vi "parse_xml.vi"(8 "error in (no error)":errorcluster, 11 "XML File Path":path) -> (0 "error out":errorcluster, 3 "raw_data []":T1(array[cluster]))   [LabVIEW 2015, in "lv-unit-conversion.lvlib"]
uses:
  lv-unit-conversion.lvlib
  _controls/error.ctl
  <vilib>/xml/Load XML File.vi
  <vilib>/xml/Close Reference(Node).vi
  <vilib>/xml/NI_XML.lvlib
  <resource>/objmgr/DOMUserDefRef.rc
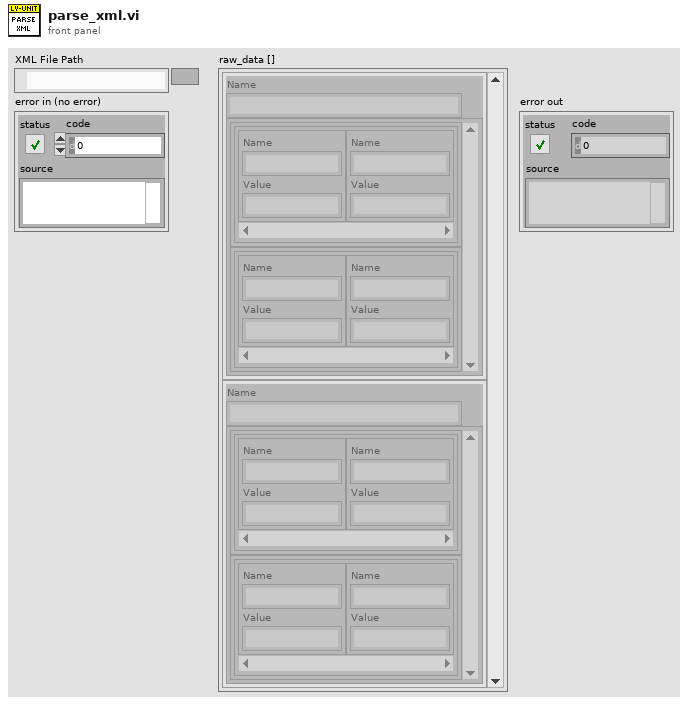
[diagram p1: front panel]
types:
  T1 = cluster{"Name":string, cluster{cluster{"Name":string, "Value":string}[]}[]}[]
  T2 = typedef "lv-unit-conversion.lvlib/error.ctl" = enum16{"<lv-unit-conversion_error>", "unit_not_found", "xml_parser", "<null>"}
  T3 = cluster{cluster{"Name":string, "Value":string}[]}
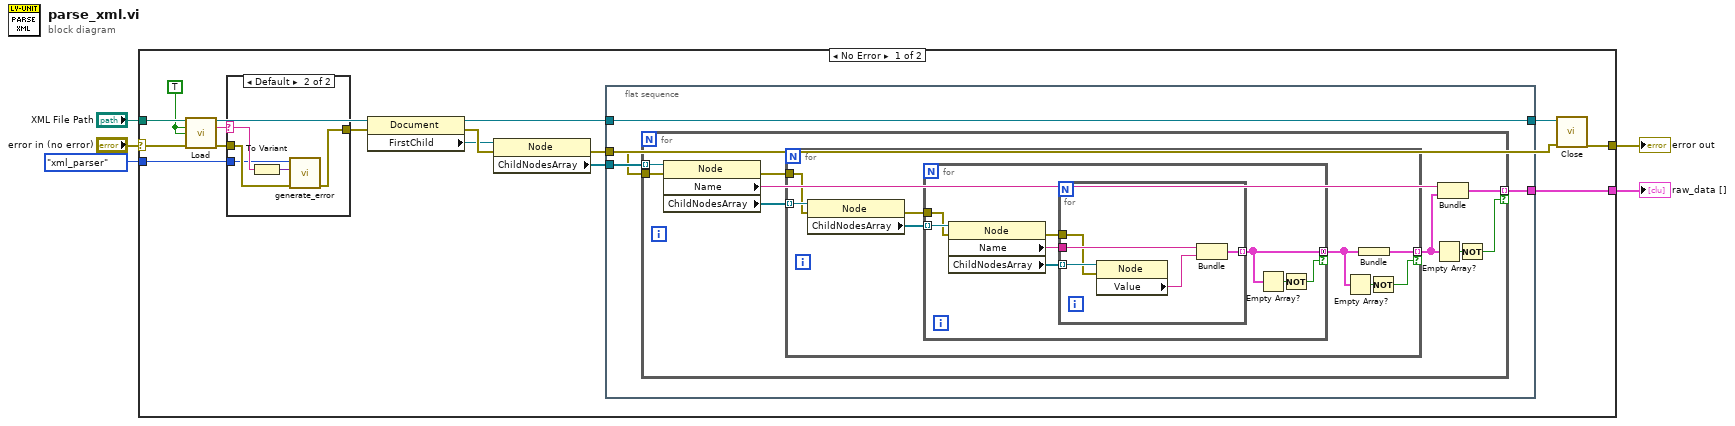
[diagram p0: block diagram]
diagram:
  n1 = case shown="No Error" "error in (no error)" {
    selector: "error in (no error)" -> [w10 w62]
    tunnel: "XML File Path" -> [w21 _]
    tunnel: [w15 _] -> w4
    tunnel: [w12 w62] -> w3
    tunnel: error."xml_parser" ("error") -> [w6 _]
    frame No Error {
      w20 = TRUE ("process namespaces (False)")
      n2 = call-poly <vilib>:"Load.vi"("path to XML document"=w21, "process namespaces (False)"=w20, "process schema (False)"=w20, "error in (no error)"=w10) -> ("DOM document out"=w19:refnum<k20>, "parse errors"=w9:string, "error out"=w8:errorcluster)  [unwired: 9 in]
      n3 = case shown="Default" w9 {
        selector: w9 -> [_ w27]
        tunnel: w8 -> [w22 w26]
        tunnel: [w22 w25] -> w7
        tunnel: w6 -> [_ w24]
        frame "" {
        }
        frame Default {
          n4 = To Variant(anything=w27) -> (Variant=w23:variant)
          n5 = call "generate_error.vi"("error in (no error)"=w26, "data"=w23, "error"=w24) -> ("error out"=w25:errorcluster)  [unwired: 8 in]
        }
      }
      n6 = property class="Document"(reference=w19, error in=w7) -> (reference out=w14:refnum<k20>, error out=w17:errorcluster, "FirstChild"=w16:refnum<k20>)
      n7 = property class="Node"(reference=w16, error in=w17) -> (error out=w11:errorcluster, "ChildNodesArray"=w18:refnum<k20>[])  [unwired: 1 out]
      n8 = flat-sequence {
        tunnel: w18 -> [w31]
        tunnel: [w30] -> w15
        tunnel: w14 -> [w29]
        tunnel: [w29] -> w13
        tunnel: w11 -> [w28]
        frame #0 {
          n9 = for {
            tunnel: w31 -> [w40] mode=indexing
            tunnel: [w39] -> w30 mode=indexing if=w36
            tunnel: w28 -> [w35]
            n10 = property class="Node"(reference=w40, error in=w35) -> (error out=w32:errorcluster, "Name"=w33:string, "ChildNodesArray"=w34:refnum<k20>[])  [unwired: 1 out]
            n11 = for {
              tunnel: w34 -> [w48] mode=indexing
              tunnel: [w44] -> w37 mode=indexing if=w45
              tunnel: w32 -> [w42]
              n12 = property class="Node"(reference=w48, error in=w42) -> (error out=w41:errorcluster, "ChildNodesArray"=w47:refnum<k20>[])  [unwired: 1 out]
              n13 = for {
                tunnel: w47 -> [w56] mode=indexing
                tunnel: [w52] -> w43 mode=concatenating if=w51
                tunnel: w41 -> [w50]
                n14 = property class="Node"(reference=w56, error in=w50) -> (error out=w49:errorcluster, "Name"=w54:string, "ChildNodesArray"=w55:refnum<k20>[])  [unwired: 1 out]
                n15 = for {
                  tunnel: w55 -> [w61] mode=indexing
                  tunnel: w54 -> [w58]
                  tunnel: [w59] -> w52 mode=indexing
                  tunnel: w49 -> [w57]
                  n16 = property class="Node"(reference=w61, error in=w57) -> ("Value"=w60:string)  [unwired: 2 out]
                  n17 = Bundle("Name"=w58, "Value"=w60) -> (w59:cluster{"Name":string, "Value":string})  [unwired: 1 in]
                }
                n18 = Empty Array?(array=w52) -> (empty?=w53:bool)
                n19 = Not(x=w53) -> (.not. x?=w51:bool)
              }
              n20 = Empty Array?(array=w43) -> (empty?=w46:bool)
              n21 = Bundle(w43) -> (w44:T3)  [unwired: 1 in]
              n22 = Not(x=w46) -> (.not. x?=w45:bool)
            }
            n23 = Empty Array?(array=w37) -> (empty?=w38:bool)
            n24 = Bundle("Name"=w33, w37) -> (w39:cluster{"Name":string, cluster{cluster[]}[]})  [unwired: 1 in]
            n25 = Not(x=w38) -> (.not. x?=w36:bool)
          }
        }
      }
      n26 = call-poly <vilib>:"Close.vi"("error in (no error)"=w11, "node"=w13) -> ("error out"=w12:errorcluster)  [unwired: 7 in]
    }
    frame Error {
    }
  }
  "raw_data []" <- w4
  "error out" <- w3
